vi "Configure Pattern Condition.vi"(8 "Delta Time (2.5E-9)":dbl=2.5e-09, 9 "Trigger Condition (0: True)":u16(ring) items=["True", "False", "Less Than", "More Than", "Equal", "Not Equal"], 10 "Clock Source (0: Channel 1)":u16(ring) items=["Channel 1"=0, "Channel 2"=1, "Channel 3"=2, "Channel 4"=3, "None"=8], 11 "Input Command String":string) -> (1 "Output Command String":string)   [LabVIEW 2013, in "Tektronix DPO MSO 2000 4000 Series.lvlib"]
doc: "Configures pattern condition settings inside logic trigger."
uses:
  Tektronix DPO MSO 2000 4000 Series.lvlib
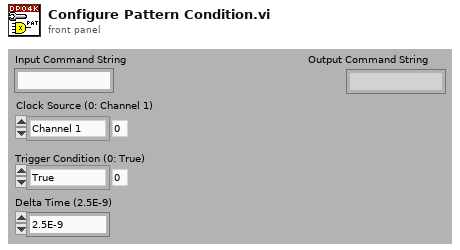
[diagram p1: front panel]
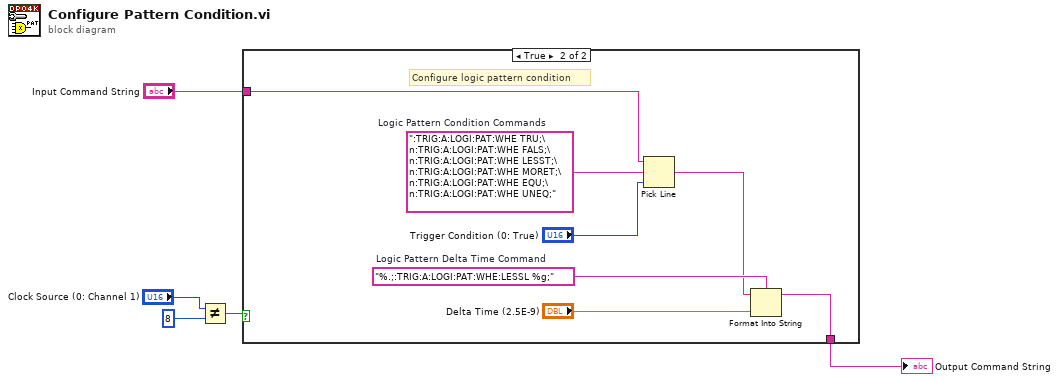
[diagram p0: block diagram]
diagram:
  n1 = Not Equal?(x="Clock Source (0: Channel 1)", y=8) -> (x != y?=w4:bool)
  n2 = case shown="True" w4 {
    tunnel: "Input Command String" -> [w6 w8]
    tunnel: [w6 w9] -> w2
    frame False {
      # "None clock source"
    }
    frame True {
      w11 = "%.;:TRIG:A:LOGI:PAT:WHE:LESSL %g;"  # Logic Pattern Delta Time Command
      w13 = ":TRIG:A:LOGI:PAT:WHE TRU;\n:TRIG:A:LOGI:PAT:WHE FALS;\n:TRIG:A:LOGI:PAT:WHE LESST;\n:TRIG:A:LOGI:PAT:WHE MORET;\n:TRIG:A:LOGI:PAT:WHE EQU;\n:TRIG:A:LOGI:PAT:WHE UNEQ;"  # Logic Pattern Condition Commands
      # "Configure logic pattern condition"
      n3 = Pick Line(string ("")=w8, multi-line string=w13, line index="Trigger Condition (0: True)") -> (output string=w10:string)
      n4 = Format Into String(format string=w11, initial string=w10, "Delta Time (2.5E-9)") -> (resulting string=w9:string)  [unwired: 1 in, 1 out]
    }
  }
  "Output Command String" <- w2
